vi "SSP - get cluster detailst.vi"(8 "error in (no error)":errorcluster, 11 "JSON string":string) -> (0 "error out":errorcluster, 3 "value":string)   [LabVIEW 2020, in "ui-testing.lvlib"]
doc: "copyright: Thomas Zilliox©"
uses:
  ui-testing.lvlib
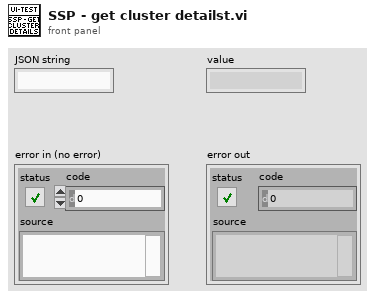
[diagram p1: front panel]
types:
  T1 = cluster{"control":string, "subpanel":string, "subsubpanel":string}
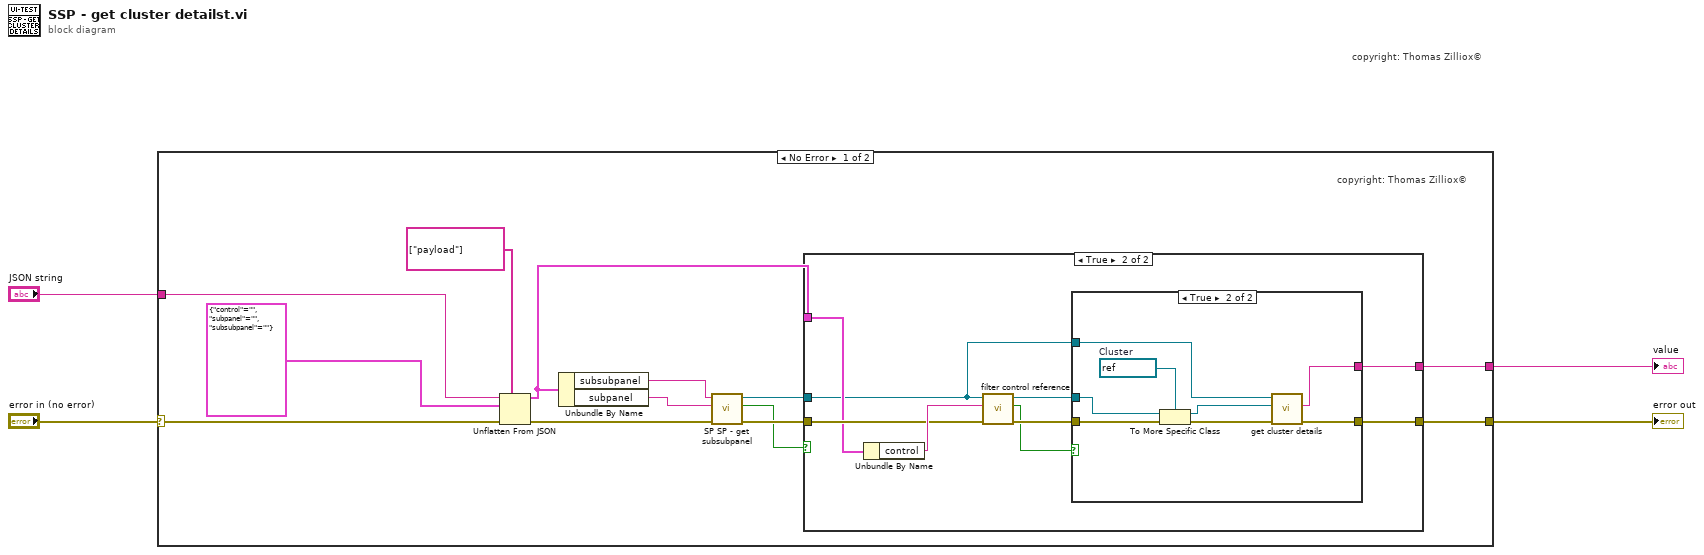
[diagram p0: block diagram]
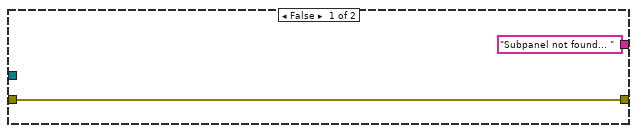
[diagram p2: hidden frame]
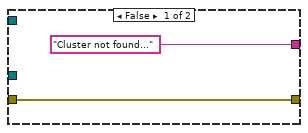
[diagram p3: hidden frame]
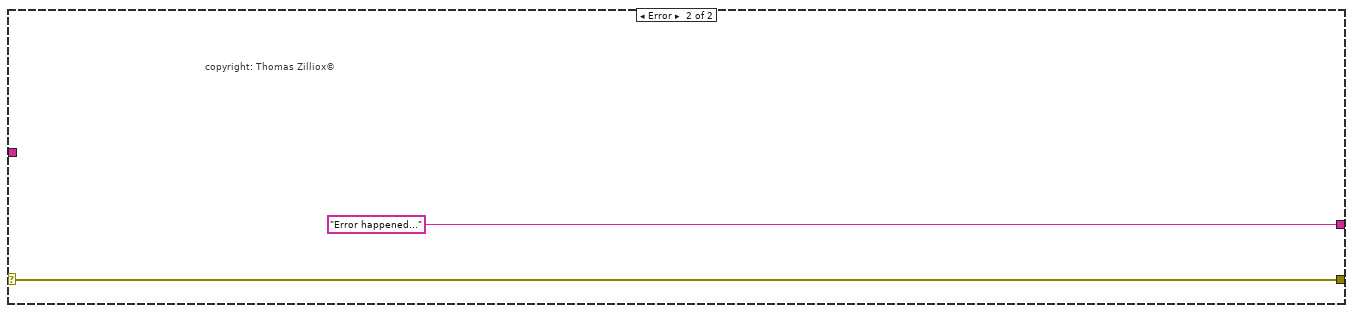
[diagram p4: hidden frame]
diagram:
  # "copyright: Thomas Zilliox©"
  n1 = case shown="No Error" "error in (no error)" {
    selector: "error in (no error)" -> [w15 w40]
    tunnel: "JSON string" -> [w16 _]
    tunnel: [w12 w40] -> w3
    tunnel: [w13 "Error happened..."] -> w2
    frame No Error {
      # "copyright: Thomas Zilliox©"
      n2 = Unflatten From JSON(path=string[] ["payload"], JSON string=w16, type and defaults=T1 {"control"="", "subpanel"="", "subsubpanel"=""}, error in (no error)=w15) -> (value=w11:T1, error out=w8:errorcluster)  [unwired: 3 in]
      n3 = Unbundle By Name(w11) -> ("subsubpanel"=w10:string, "subpanel"=w9:string)
      n4 = call "SP SP - get subsubpanel.vi"("error in (no error)"=w8, "subpanel"=w9, "subsubpanel"=w10) -> ("error out"=w6:errorcluster, "SubSubPanel found"=w5:bool, "SubSubPanel VI"=w7:refnum<vi>)  [unwired: 5 in, 1 out]
      n5 = case shown="True" w5 {
        tunnel: ["Subpanel not found... " ("result string") w24] -> w13
        tunnel: [w18 w23] -> w12
        tunnel: w6 -> [w18 w22]
        tunnel: w7 -> [_ w20]
        tunnel: w11 -> [_ w21]
        frame False {
        }
        frame True {
          n6 = Unbundle By Name(w21) -> ("control"=w28:string)
          n7 = call "filter control reference.vi"("error in (no error)"=w22, "Control label"=w28, "VI (Caller)"=w20) -> ("error out"=w26:errorcluster, "Control found"=w25:bool, "Control ref"=w27:refnum<vi>)  [unwired: 6 in]
          n8 = case shown="True" w25 {
            tunnel: w27 -> [_ w37]
            tunnel: w26 -> [w30 w38]
            tunnel: [w30 w31] -> w23
            tunnel: ["Cluster not found..." w33] -> w24
            tunnel: w20 -> [_ w34]
            frame False {
            }
            frame True {
              w36 = refnum<vi> refnum  # Cluster
              n9 = To More Specific Class(target class=w36, reference=w37, error in=w38) -> (specific class reference=w35:refnum<vi>, error out=w32:errorcluster)
              n10 = call "get cluster details.vi"("error in"=w32, "Cluster-target"=w35, "VI Refnum"=w34) -> ("error out"=w31:errorcluster, "Control details"=w33:string)  [unwired: 7 in]
            }
          }
        }
      }
    }
    frame Error {
      # "copyright: Thomas Zilliox©"
    }
  }
  "error out" <- w3
  "value" <- w2
